vi "Create Test Suite (BrokenTests).vi.vi"(5 "Interactive (T)":bool=TRUE, 7 "Verbose (F)":bool, 8 "error in (no error)":errorcluster, 9 "Test Report":refnum<class "Test Report.lvclass">, 11 "Test Folder (default: test case defined folder)":path) -> (0 "error out":errorcluster, 3 "Test Runner.BrokenTests":refnum<class "Test Runner.BrokenTest.lvclass">)   [LabVIEW 2020, in "Test Runner.BrokenTest.lvclass"]
uses:
  Test Runner.BrokenTest.lvclass
  C:/projects/caraya/src/classes/Test Runner.Folder/Test Runner.Folder.lvclass
  classes/Test Report/Test Report.lvclass
  classes/Test Runner.Folder/Test Runner.Folder.lvclass
panel:
  out "appended path":path
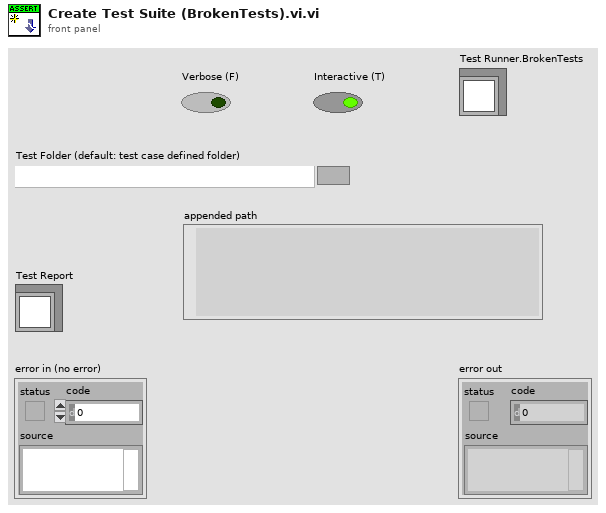
[diagram p1: front panel]
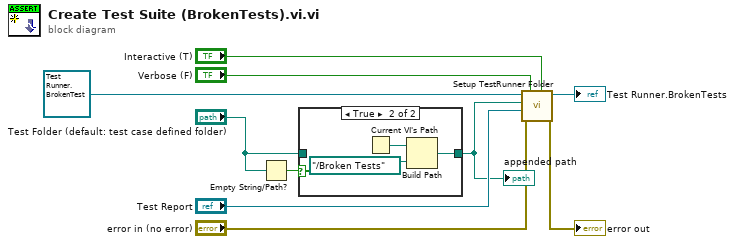
[diagram p0: block diagram]
diagram:
  n1 = Empty String/Path?(string/path="Test Folder (default: test case defined folder)") -> (empty?=w3:bool)
  n2 = case shown="True" w3 {
    tunnel: [w11 w12] -> w2
    tunnel: "Test Folder (default: test case defined folder)" -> [w11 _]
    frame False {
    }
    frame True {
      n3 = Current VI's Path() -> (path=w14:path)
      n4 = Build Path(base path=w14, name or relative path=path "../Broken Tests" ("path")) -> (appended path=w12:path)
    }
  }
  "appended path" <- w2
  n5 = call "Setup TestRunner Folder.vi"("Interactive (T)"="Interactive (T)", "Verbose (F)"="Verbose (F)", "error in (no error)"="error in (no error)", "Test Report"="Test Report", "Directory to search"=w2, "Test Runner.Folder"=refnum<class "Test Runner.BrokenTest.lvclass"> refnum ("Test Runner.BrokenTests in")) -> ("error out"=→"error out":errorcluster, "Test Runner.Folder out"=→"Test Runner.BrokenTests":refnum<class "Test Runner.BrokenTest.lvclass">)  [unwired: 4 in]
